vi "Payload to Real.vi"(3 "Payload":string) -> (1 "Real":dbl[](array[numeric]))   [LabVIEW 2019]
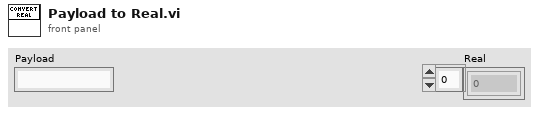
[diagram p1: front panel]
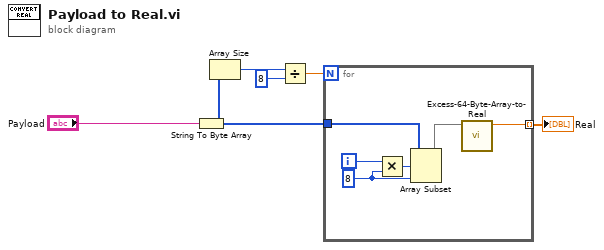
[diagram p0: block diagram]
diagram:
  n1 = String To Byte Array(string="Payload") -> (unsigned byte array=w3:u8[])
  n2 = Array Size(array=w3) -> (size(s)=w6:i32)
  n3 = Divide(x=w6, y=8) -> (x/y=w4:dbl)
  n4 = for {
    N: w4 -> [_]
    tunnel: w3 -> [w8]
    tunnel: [w7] -> w1 mode=indexing
    i -> [w12]
    w9 = 8 ("y")
    n5 = Multiply(x=w12, y=w9) -> (x*y=w10:i32)
    n6 = Array Subset(array=w8, index=w10, length=w9) -> (w11:u8[])
    n7 = call "Excess-64-Byte-Array-to-Real.vi"("Byte array (4 or 8 bytes)"=w11) -> ("Real Number"=w7:dbl)  [unwired: 10 in]
  }
  "Real" <- w1
